vi "Process data.vi"(8 "error in (no error)":errorcluster, 10 "input array":dbl[][](array[numeric]), 11 "ExampleClassDKaleidoscope in":refnum<class "ExampleClassDMath.lvclass">) -> (0 "error out":errorcluster, 2 "output array":dbl[][](array[numeric]), 3 "ExampleClassDKaleidoscope out":refnum<class "ExampleClassDMath.lvclass">)   [LabVIEW 2012, in "ExampleClassDMath.lvclass"]
uses:
  ExampleClassDMath.lvclass
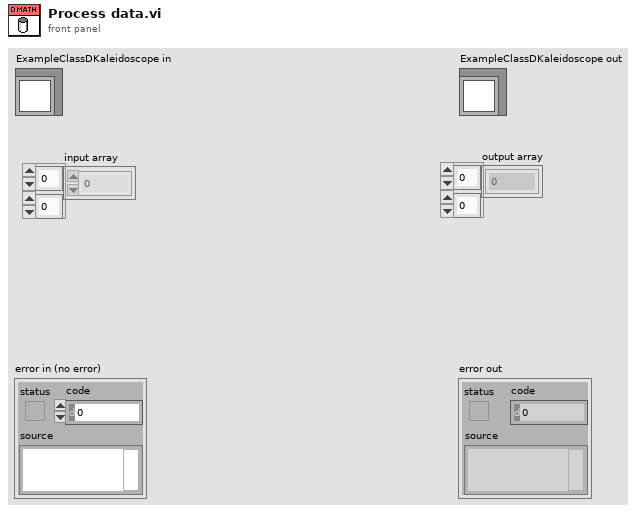
[diagram p1: front panel]
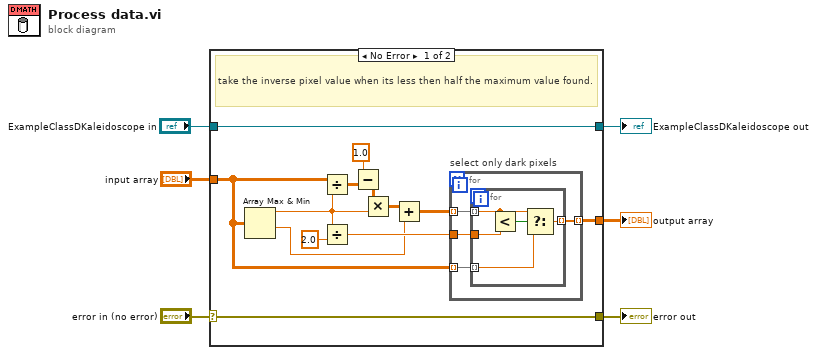
[diagram p0: block diagram]
diagram:
  n1 = case shown="No Error" "error in (no error)" {
    selector: "error in (no error)" -> [w8 w29]
    tunnel: [w19 w30] -> w6
    tunnel: "input array" -> [w18 w30]
    tunnel: [w8 w29] -> w3
    tunnel: [w7 w31] -> w2
    tunnel: "ExampleClassDKaleidoscope in" -> [w7 w31]
    frame No Error {
      # "take the inverse pixel value when its less then half the maximum value found."
      n2 = Array Max & Min(array=w18) -> (max value=w14:dbl, min value=w11:dbl)  [unwired: 2 out]
      n3 = Divide(x=w18, y=w14) -> (x/y=w16:dbl[][])
      n4 = Divide(x=w14, y=2.0) -> (x/y=w12:dbl)
      n5 = Subtract(x=1.0, y=w16) -> (x-y=w17:dbl[][])
      n6 = Multiply(x=w17, y=w14) -> (x*y=w10:dbl[][])
      n7 = Add(x=w10, y=w11) -> (x+y=w9:dbl[][])
      n8 = for "select only dark pixels" {
        tunnel: w9 -> [w23] mode=indexing
        tunnel: w12 -> [w22]
        tunnel: [w21] -> w19 mode=indexing
        tunnel: w18 -> [w20] mode=indexing
        n9 = for {
          tunnel: w23 -> [w25] mode=indexing
          tunnel: w22 -> [w28]
          tunnel: [w26] -> w21 mode=indexing
          tunnel: w20 -> [w24] mode=indexing
          n10 = Less?(x=w25, y=w28) -> (x < y?=w27:bool)
          n11 = Select(t=w25, s=w27, f=w24) -> (s? t:f=w26:dbl)
        }
      }
    }
    frame Error {
    }
  }
  "error out" <- w3
  "ExampleClassDKaleidoscope out" <- w2
  "output array" <- w6
